vi "STDTrue.vi"(11 "Array":dbl[][](array[numeric]) format="%#_2g") -> (0 "My std":dbl[](array[numeric]), 1 "[Xi-X]":dbl[][](array[numeric]), 2 "Xi - X":dbl[](array[numeric]), 3 "mean":dbl[](array[numeric]) format="%#_4g")   [LabVIEW 2023]
uses:
  <vilib>/Analysis/NI_AALBase.lvlib
panel:
  out "variance":dbl[](array[numeric]) format="%#_4g"
  out "My Variance":dbl[](array[numeric]) format="%#_4g"
  out "std":dbl[](array[numeric])
  out "Mean":dbl[](array[numeric]) format="%#_4g"
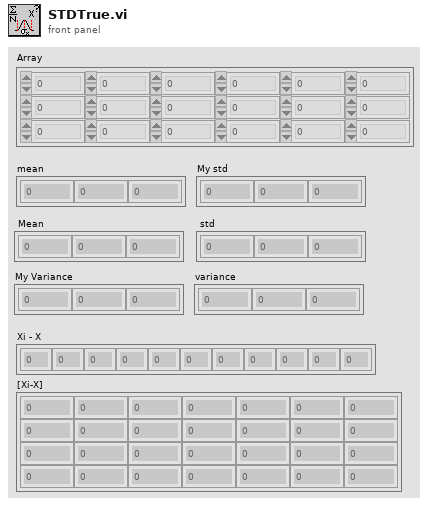
[diagram p1: front panel]
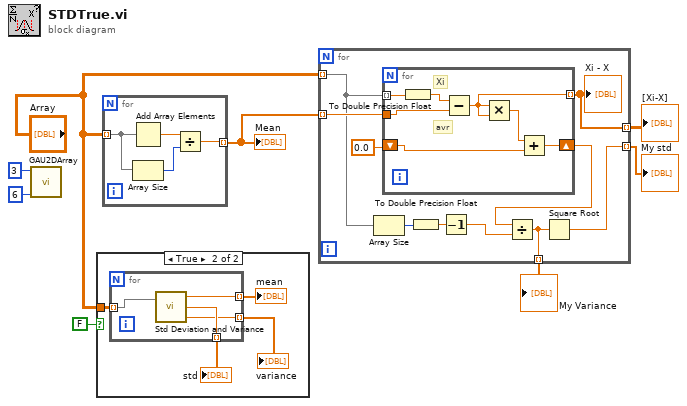
[diagram p0: block diagram]
diagram:
  n1 = call "GAU2DArray.vi"("Colums"=6, "Rows"=3) -> ()  [unwired: 7 in, 3 out]
  n2 = case shown="True" FALSE {
    tunnel: "Array" -> [_ w10]
    frame False {
    }
    frame True {
      n3 = for {
        tunnel: w10 -> [w16] mode=indexing
        tunnel: [w15] -> w12 mode=indexing
        tunnel: [w14] -> w11 mode=indexing
        tunnel: [w13] -> w9 mode=indexing
        n4 = call <vilib>:"Std Deviation and Variance.vi"("X"=w16) -> ("mean"=w15:dbl, "standard deviation"=w14:dbl, "variance"=w13:dbl)  [unwired: 1 in]
      }
      "mean" <- w12
      "std" <- w11
      "variance" <- w9
    }
  }
  n5 = for {
    tunnel: "Array" -> [w18] mode=indexing
    tunnel: [w17] -> w6 mode=indexing
    n6 = Add Array Elements(numeric array=w18) -> (sum=w20:dbl)
    n7 = Array Size(array=w18) -> (size(s)=w19:i32)
    n8 = Divide(x=w20, y=w19) -> (x/y=w17:dbl)
  }
  "Mean" <- w6
  n9 = for {
    tunnel: "Array" -> [w28] mode=indexing
    tunnel: w6 -> [w30] mode=indexing
    tunnel: [w26] -> w5 mode=indexing
    tunnel: [w22] -> w3 mode=indexing
    tunnel: [w21] -> w1 mode=indexing
    n10 = Array Size(array=w28) -> (size(s)=w27:i32)
    n11 = for {
      tunnel: w28 -> [w36] mode=indexing
      tunnel: w30 -> [w37]
      shift-right: [w32] -> w23
      shift-left: 0.0 -> [w33]
      tunnel: [w31] -> w21 mode=indexing
      # "Xi"
      # "avr"
      n12 = To Double Precision Float(number=w36) -> (double precision float=w35:dbl)
      n13 = Subtract(x=w35, y=w37) -> (x-y=w31:dbl)
      n14 = Multiply(x=w31, y=w31) -> (x*y=w34:dbl)
      n15 = Add(x=w34, y=w33) -> (x+y=w32:dbl)
    }
    "Xi - X" <- w21
    n16 = To Double Precision Float(number=w27) -> (double precision float=w25:dbl)
    n17 = Decrement(x=w25) -> (x-1=w24:dbl)
    n18 = Divide(x=w23, y=w24) -> (x/y=w22:dbl)
    n19 = Square Root(x=w22) -> (sqrt(x)=w26:dbl)
  }
  "My std" <- w5
  "My Variance" <- w3
  "[Xi-X]" <- w1
